vi "Init Data.vi"(10 "Data":T1) -> (3 "Msg out":refnum<class "Msg.lvclass">)   [LabVIEW 2020, in "SyncTicks.lvlib" / "Msg.lvclass"]
uses:
  Msg.lvclass
  Data.ctl
  SyncTicks.lvlib
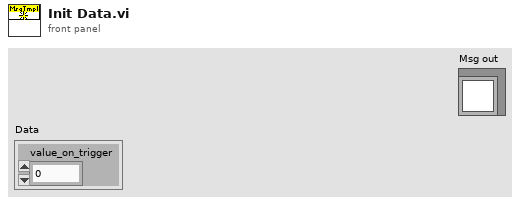
[diagram p1: front panel]
types:
  T1 = typedef "SyncTicks.lvlib/Data.ctl" = cluster{"value_on_trigger":u32}
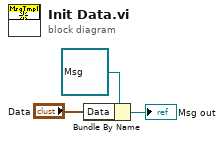
[diagram p0: block diagram]
diagram:
  n1 = Bundle By Name(cluster=refnum<class "Msg.lvclass"> refnum ("Msg out"), "Data"="Data") -> (→"Msg out":refnum<class "Msg.lvclass">)
